vi "Toggle.vi"() -> ()   [LabVIEW 2017]
panel:
  out "output":bool
  in  "toggle?":bool
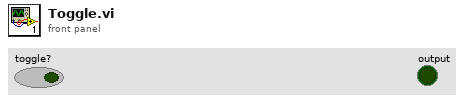
[diagram p1: front panel]
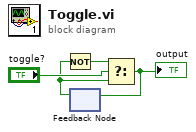
[diagram p0: block diagram]
diagram:
  n1 = feedback #1() -> (w1:bool)  [unwired: 1 in]
  n2 = Not(x=w1) -> (.not. x?=w4:bool)
  n3 = Select(t=w4, s="toggle?", f=w1) -> (s? t:f=w2:bool)
  "output" <- w2
  n4 = feedback-in #1(w2) -> ()
